vi "Concatenate Field Names.vi"(1 "B":string, 2 "A":string) -> (0 "field name":string)   [LabVIEW 2020, in "PV Access.lvlib" / "PV Data.lvlib"]
uses:
  PV Data.lvlib
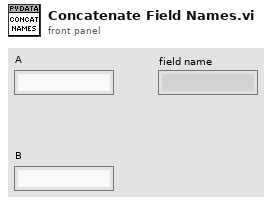
[diagram p1: front panel]
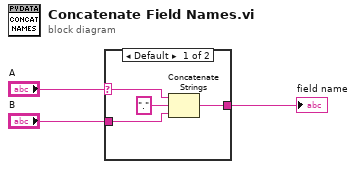
[diagram p0: block diagram]
diagram:
  n1 = case shown="Default" "A" {
    selector: "A" -> [w7 _]
    tunnel: [w4 w8] -> w1
    tunnel: "B" -> [w6 w8]
    frame Default {
      n2 = Concatenate Strings(w7, "." ("string"), w6) -> (w4:string)
    }
    frame "" {
    }
  }
  "field name" <- w1
